vi "exec.vi"(8 "error in (no error)":errorcluster, 10 "context":refnum<class "Context.lvclass">, 11 "SendOutputData in":refnum<class "SendOutputData.lvclass">) -> (0 "error out":errorcluster, 2 "context 2":refnum<class "Context.lvclass">, 3 "SendOutputData out":refnum<class "SendOutputData.lvclass">)   [LabVIEW 2013, in "SendOutputData.lvclass"]
uses:
  SendOutputData.lvclass
  Context/Context.lvclass
  SendOutputData.lvclass/SendOutputData.ctl
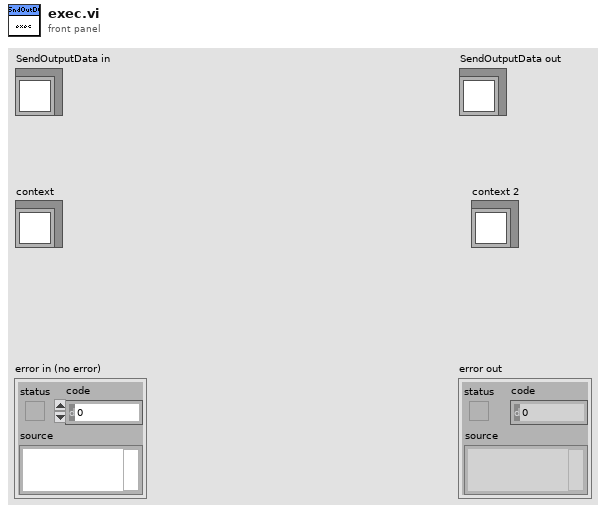
[diagram p1: front panel]
types:
  T1 = typedef "ILCCommon.lvlib/ILCTypedefs.lvlib/OutputData.ctl" = cluster{"Step & Direction":i16, "Blower RPM":u8, "PWM (SSR)":u8, "Ch1":u16, "Ch2":u16, "Ch3":u16, "Ch4":u16}
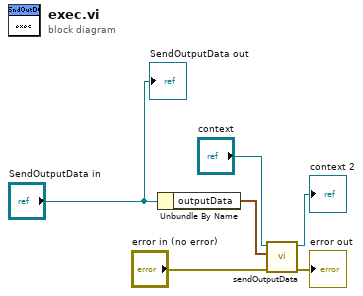
[diagram p0: block diagram]
diagram:
  n1 = Unbundle By Name("SendOutputData in") -> ("outputData"=w1:T1)
  n2 = call "sendOutputData.vi"("error in (no error)"="error in (no error)", "outputData"=w1, "Context in"="context") -> ("error out"=→"error out":errorcluster, "Context out"=→"context 2":refnum<class "Context.lvclass">)  [unwired: 7 in]
  "SendOutputData out" <- "SendOutputData in"
